vi "Read.vi"(8 "error in (no error)":errorcluster, 11 "NI DMM in":refnum<class "NI DMM.lvclass">) -> (0 "error out":errorcluster, 3 "NI DMM out":refnum<class "NI DMM.lvclass">)   [LabVIEW 2020, in "NI DMM.lvclass"]
uses:
  NI DMM.lvclass
  D:/Users/Marco Yang/Downloads/LVOOP 2012/LVOOP 2012/DMM/DMM.lvclass
  NI DMM.lvclass/NI DMM.ctl
  DMM/DMM.lvclass/DMM.ctl
  DMM/DMM.lvclass
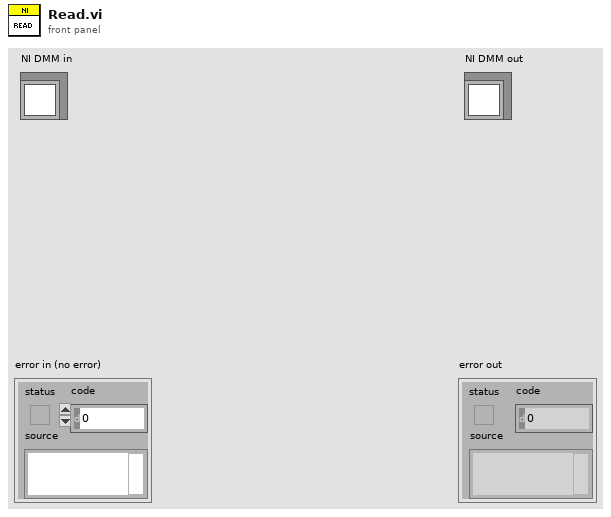
[diagram p1: front panel]
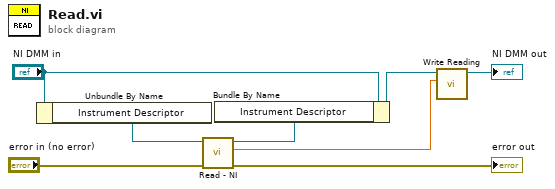
[diagram p0: block diagram]
diagram:
  n1 = Unbundle By Name("NI DMM in") -> ("Instrument Descriptor"=w6:refnum<k15>)
  n2 = call "Read - NI.vi"("error in (no error)"="error in (no error)", "instrument handle"=w6) -> ("error out"=→"error out":errorcluster, "Measurement"=w1:dbl, "instrument handle out"=w5:refnum<k15>)  [unwired: 7 in]
  n3 = Bundle By Name(cluster="NI DMM in", "Instrument Descriptor"=w5) -> (w3:refnum<class "NI DMM.lvclass">)
  n4 = call "Write Reading.vi"("Reading"=w1, "DMM in"=w3) -> ("DMM out"=→"NI DMM out":refnum<class "NI DMM.lvclass">)  [unwired: 8 in, 1 out]
